vi "Send.vi"(8 "Error In":errorcluster, 9 "Colleague":refnum<class "Colleague.lvclass">, 10 "Message":string, 11 "reference in":refnum<class "ManagerMediator.lvclass">) -> (0 "Error Out":errorcluster, 3 "reference in":refnum<class "ManagerMediator.lvclass">)   [LabVIEW 2020, in "ManagerMediator.lvclass"]
uses:
  ManagerMediator.lvclass
  Colleague_class/Colleague.lvclass
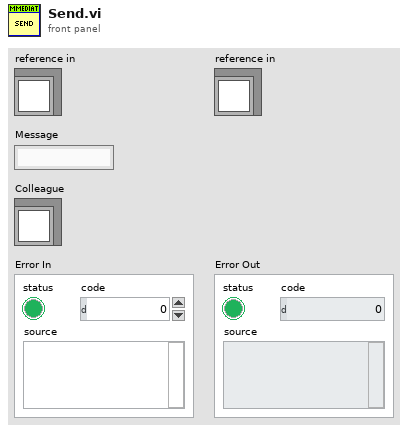
[diagram p1: front panel]
types:
  T1 = typedef "ManagerMediator.lvclass/ObjectAttributes.ctl" = cluster{"Customer":refnum<class "Colleague.lvclass">, "Programmer":refnum<class "Colleague.lvclass">, "Tester":refnum<class "Colleague.lvclass">}
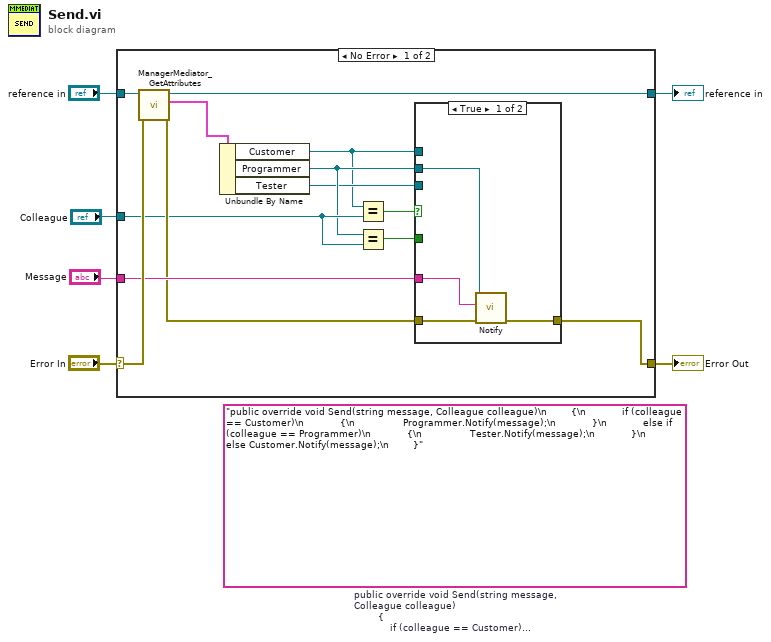
[diagram p0: block diagram]
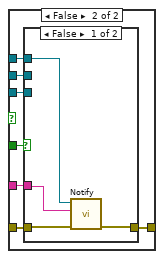
[diagram p2: hidden frame]
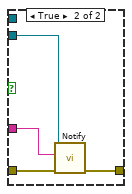
[diagram p3: hidden frame]
diagram:
  (unwired) "public override void Send(string message, Colleague colleague)\n        {\n            if (colleague == Customer)\n            {\n                Programmer.Notify(message);\n            }\n            else if (colleague == Programmer)\n            {\n                Tester.Notify(message);\n            }\n            else Customer.Notify(message);\n        }"  # public override void Send(string message, Colleague colleague)         {             if (colleague == Customer)             {                 Programmer.Notify(message);             }             else if (colleague == Programmer)             {                 Tester.Notify(message);             }             else Customer.Notify(message);         }
  n1 = case shown="No Error" "Error In" {
    selector: "Error In" -> [w18 w40]
    tunnel: [w13 w40] -> w5
    tunnel: [w17 w39] -> w3
    tunnel: "reference in" -> [w19 w39]
    tunnel: "Colleague" -> [w11 _]
    tunnel: "Message" -> [w15 _]
    frame No Error {
      n2 = call "ManagerMediator_GetAttributes.vi"("error in (no error)"=w18, "reference in"=w19) -> ("error out"=w14:errorcluster, "Data"=w16:T1, "reference out"=w17:refnum<class "ManagerMediator.lvclass">)  [unwired: 6 in, 1 out]
      n3 = Unbundle By Name(w16) -> ("Customer"=w7:refnum<class "Colleague.lvclass">, "Programmer"=w10:refnum<class "Colleague.lvclass">, "Tester"=w8:refnum<class "Colleague.lvclass">)
      n4 = Equal?(x=w7, y=w11) -> (x = y?=w12:bool)
      n5 = Equal?(x=w10, y=w11) -> (x = y?=w9:bool)
      n6 = case shown="True" w12 {
        tunnel: w10 -> [w23 w30]
        tunnel: w15 -> [w22 w29]
        tunnel: w14 -> [w21 w28]
        tunnel: [w20 w27] -> w13
        tunnel: w9 -> [_ w26]
        tunnel: w8 -> [_ w25]
        tunnel: w7 -> [_ w24]
        frame True {
          n7 = call-dynamic "Notify.vi"("Error In"=w21, "Message"=w22, "reference in"=w23) -> ("Error Out"=w20:errorcluster)  [unwired: 7 in, 1 out]
        }
        frame False {
          n8 = case shown="False" w26 {
            tunnel: w30 -> [_ _]
            tunnel: w29 -> [w31 w38]
            tunnel: w28 -> [w34 w37]
            tunnel: [w33 w36] -> w27
            tunnel: w25 -> [_ w35]
            tunnel: w24 -> [w32 _]
            frame False {
              n9 = call-dynamic "Notify.vi"("Error In"=w34, "Message"=w31, "reference in"=w32) -> ("Error Out"=w33:errorcluster)  [unwired: 7 in, 1 out]
            }
            frame True {
              n10 = call-dynamic "Notify.vi"("Error In"=w37, "Message"=w38, "reference in"=w35) -> ("Error Out"=w36:errorcluster)  [unwired: 7 in, 1 out]
            }
          }
        }
      }
    }
    frame Error {
    }
  }
  "Error Out" <- w5
  "reference in" <- w3
